vi "BELKIN EAGLE RT Main V2.vi"() -> ()   [LabVIEW 2015]
uses:
  <vilib>/vision/Image Controls.llb/IMAQ Image.ctl
  <vilib>/userdefined/High Color/IMAQdx.ctl
  Controls/BELKIN RT State.ctl
  IP results.ctl
  Controls/Command Typedef.ctl
  Stream/Controls/RT Streamer Queue element.ctl
  Stream/Controls/RT Streamer State.ctl
  Stream/LP Globals.vi
  <vilib>/FPGAPlugInAG/cRIO-9030/niLvFpga_Open_cRIO-9030.vi
  <vilib>/rvi/interface/common/dynamic/niFpgaDynamicAddResources.vi
  <vilib>/FPGAPlugInAG/Dynamic/niLvFpga_Abort_Dynamic.vi
  <vilib>/FPGAPlugInAG/Dynamic/niLvFpga_Reset_Dynamic.vi
  <vilib>/FPGAPlugInAG/Dynamic/niLvFpga_Run_Dynamic.vi
  <vilib>/Utility/error.llb/Error Cluster From Error Code.vi
  <vilib>/rvi/interface/common/niFpgaWaitOnOcc.vi
  <vilib>/rvi/errors/niLvFpgaAdjustHostInterfaceError.vi
  <vilib>/rvi/interface/nirviOpenFPGA/nirviOpenFPGA.xnode
  FPGA Bitfiles/BELKINEAGLEGUI_FPGATarget_EagleFPGAScanner_AddXN+PC+cM.lvbitx
  RT/Eagle_FPGA Scanner Control.vi
  <vilib>/rvi/interface/nirviMethod/nirviMethod.xnode
  <vilib>/rvi/interface/nirviReadWriteControl/nirviReadWriteControl.xnode
  <vilib>/rvi/interface/Simulation/niFpgaSimulationCallBeginRW.vi
  <vilib>/vision/NI_Vision_Development_Module.lvlib
  <vilib>/rvi/errors/niLvFpgaMergeErrorWithErrorCode.vi
  <vilib>/FPGAPlugInAG/Dynamic/niLvFpga_StopFifo_Dynamic.vi
  <vilib>/FPGAPlugInAG/Dynamic/niLvFpga_ConfigureFifo_Dynamic.vi
  <vilib>/FPGAPlugInAG/Dynamic/niLvFpga_StartFifo_Dynamic.vi
  NiFpgaLv.dll
panel:
  in  "FPGA VI Reference IN":refnum<k20>
  out "RoteteImages":bool
  out "Y Points":i32[](array[numeric])
  out "X Points":i32[](array[numeric])
  in  "Threshold":u8
  out "ImageIndex":i32
  out "IP Results":T1
  out "SystemState":T2=enum."Find Limbus"
  in  "Image Dir Path":path=path "c:/Images/DariaSynthMove" caption="Image Path"
  out "Simulation":bool
  in  "CamSession":T3="cam0"
  in  "AutoBalance":bool
  in  "SetParams":bool
  in  "GuiVideoRate":u8=10
  out "FrameRate":dbl
  out "EyeImage":T4
  out "Algo Time":u32
  # "Realtime Main V2"
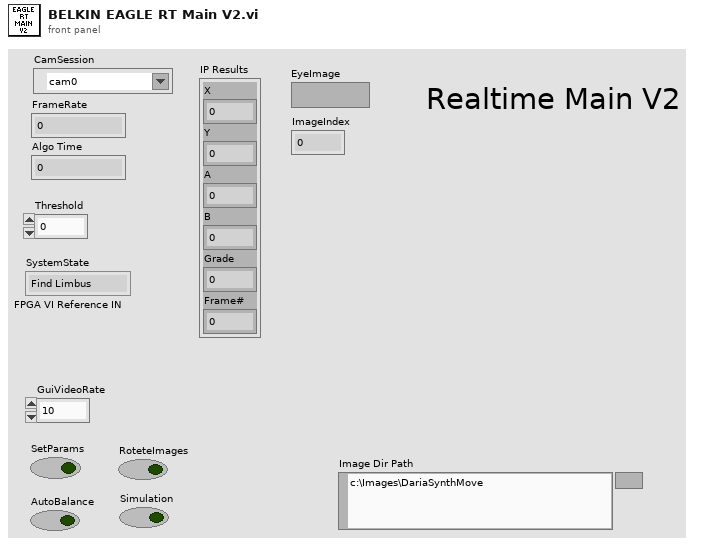
[diagram p1: front panel]
types:
  T1 = typedef "IP results.ctl" = cluster{"X":u16, "Y":u16, "A":dbl, "B":dbl, "Grade":u16, "Frame#":u16}
  T2 = typedef "BELKIN RT State.ctl" = enum16{"Initialize", "BIT", "Warm Up", "Eye Location", "Find Limbus", "Eye Track", "Fire", "Treatment Complete", "Shut Down", "Error"}
  T3 = typedef "IMAQdx.ctl" = refnum<k21>
  T4 = typedef "IMAQ Image.ctl" = refnum<image>
  T5 = typedef "Command Typedef.ctl" = cluster{"CMD":T2, "Data":variant}
  T6 = typedef "RT Streamer Queue element.ctl" = cluster{"CMD":T7, "Data":variant, "Error in":errorcluster}
  T7 = typedef "RT Streamer State.ctl" = enum16{"Init", "Idle", "Stream", "Listen", "SetRefrashRate", "SendCmdAck", "SendCmdDone", "SendSysState", "StartRecord", "Green Cordinates", "Error"}
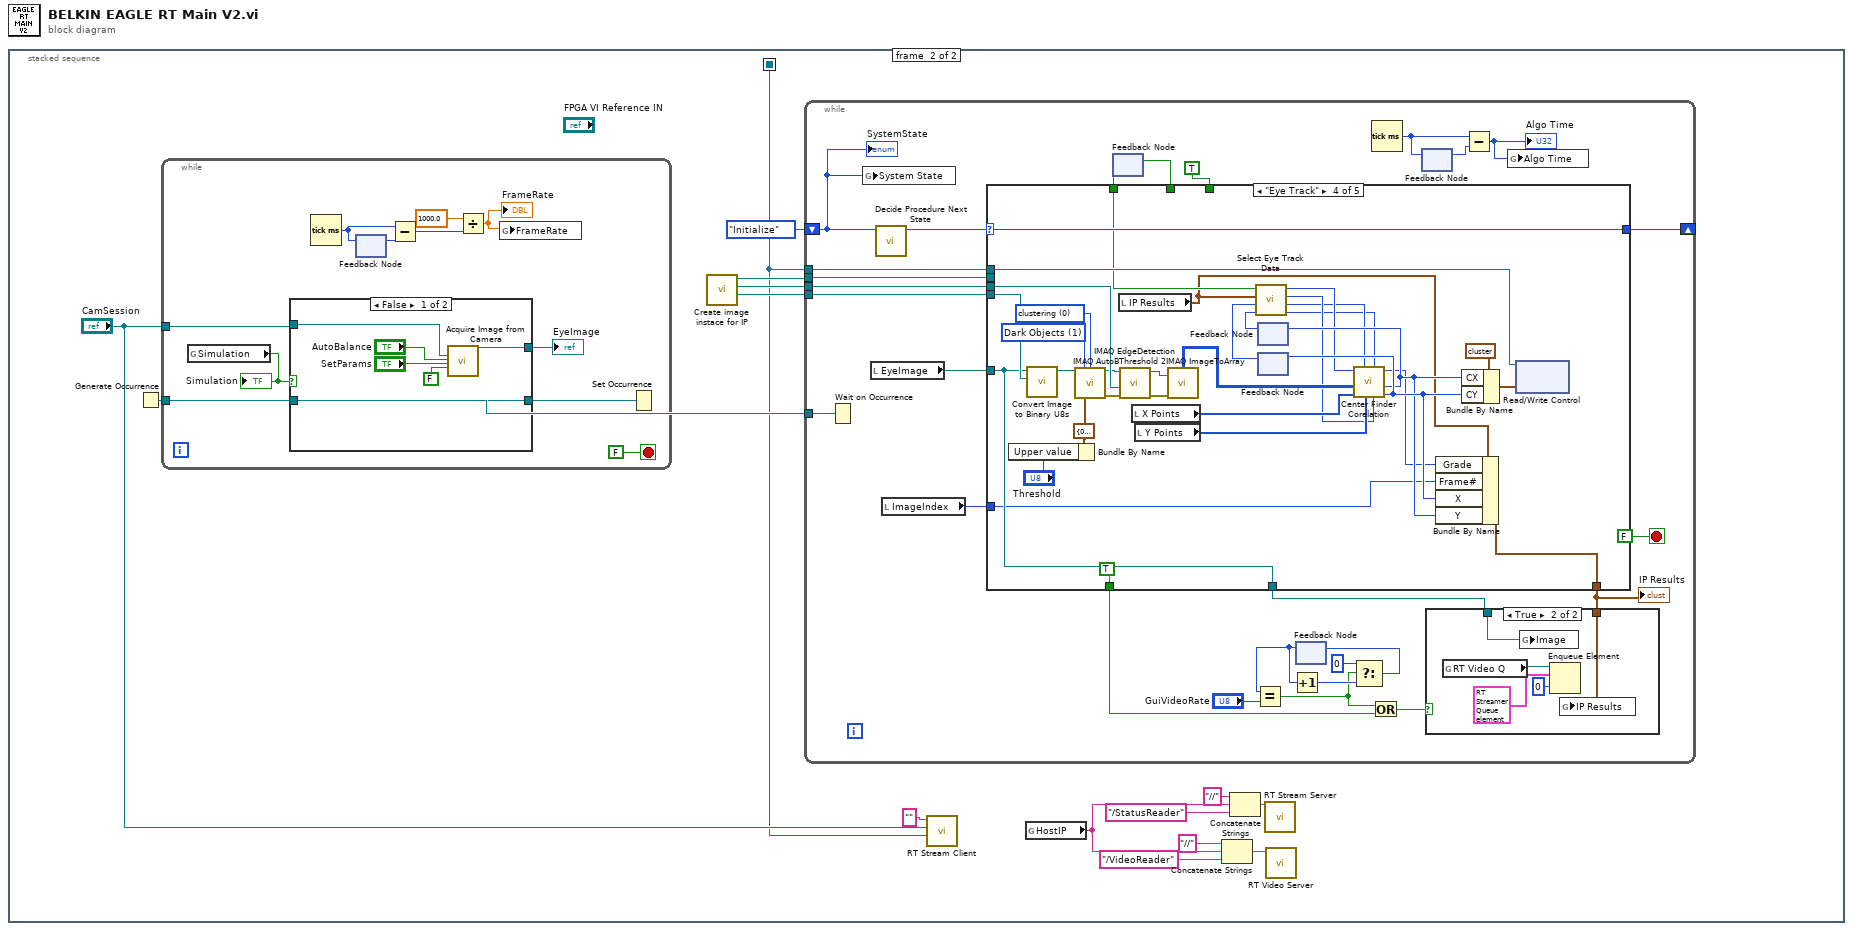
[diagram p0: block diagram]
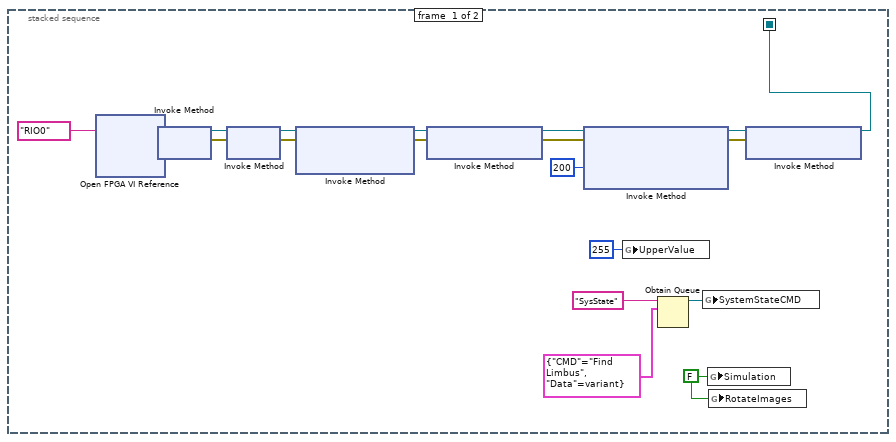
[diagram p2: hidden frame]
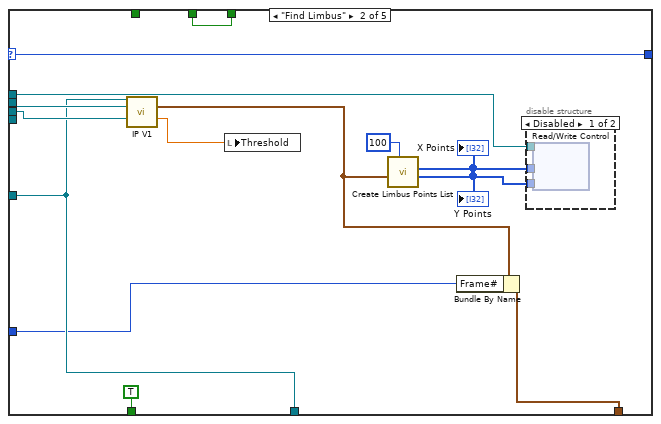
[diagram p5: hidden frame]
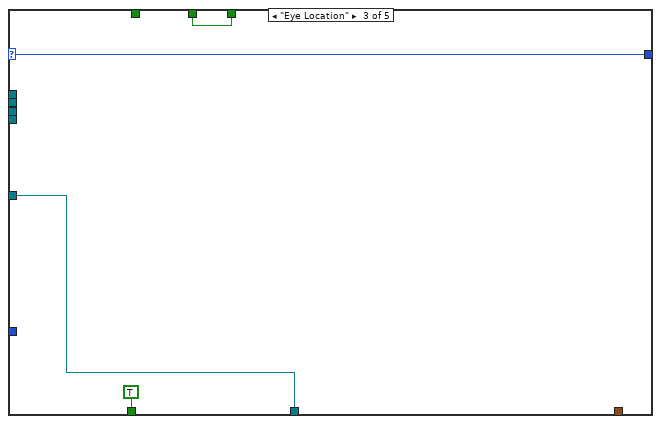
[diagram p7: hidden frame]
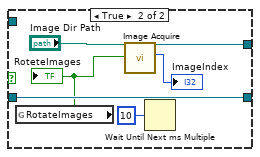
[diagram p9: hidden frame]
diagram:
  n1 = stacked-sequence {
    seq-local: [w7 _] -> [_ w21]
    frame #0 {
      w17 = FALSE ("Simulation")
      n2 = xnode "Open FPGA VI Reference"("resource name"=tag "RIO0") -> ("FPGA VI Reference Out"=w6:refnum<k20>, "error out"=w5:errorcluster)  [unwired: 1 in]
      n3 = xnode "Invoke Method"("FPGA VI Reference In"=w6, "error in"=w5) -> ("FPGA VI Reference Out"=w4:refnum<k20>, "error out"=w3:errorcluster)
      n4 = xnode "Invoke Method"("FPGA VI Reference In"=w4, "error in"=w3) -> ("FPGA VI Reference Out"=w1:refnum<k20>, "error out"=w2:errorcluster)
      n5 = xnode "Invoke Method"("FPGA VI Reference In"=w1, "error in"=w2) -> ("FPGA VI Reference Out"=w15:refnum<k20>, "error out"=w14:errorcluster)  [unwired: 1 in]
      n6 = xnode "Invoke Method"("FPGA VI Reference In"=w15, "error in"=w14) -> ("FPGA VI Reference Out"=w9:refnum<k20>, "error out"=w8:errorcluster)
      n7 = xnode "Invoke Method"("FPGA VI Reference In"=w9, "error in"=w8, "Requested Depth"=u32 200) -> ("FPGA VI Reference Out"=w11:refnum<k20>, "error out"=w10:errorcluster)  [unwired: 1 out]
      n8 = global write "LP Globals.vi" "UpperValue"(u8 255 ("UpperValue")) -> ()
      n9 = Obtain Queue(name (unnamed)="SysState", element data type=T5 {"CMD"=enum."Find Limbus", "Data"=variant}) -> (queue out=w18:refnum<queue>)  [unwired: 3 in, 2 out]
      n10 = global write "LP Globals.vi" "SystemStateCMD"(w18) -> ()
      n11 = global write "LP Globals.vi" "Simulation"(w17) -> ()
      n12 = global write "LP Globals.vi" "RotateImages"(w17) -> ()
      n13 = xnode "Invoke Method"("FPGA VI Reference In"=w11, "error in"=w10) -> ("FPGA VI Reference Out"=w7:refnum<k20>)  [unwired: 1 out]
    }
    frame #1 {
      n14 = Generate Occurrence() -> (w26:refnum<k4>)
      n15 = while {
        tunnel: "CamSession" -> [w132]
        tunnel: w26 -> [w131]
        stop <- FALSE stop-if-true
        n16 = global read "LP Globals.vi" "Simulation"() -> (w127:bool)
        "Simulation" <- w127
        n17 = case shown="False" w127 {
          tunnel: w132 -> [w143 _]
          tunnel: [w142 w149] -> w129
          tunnel: w131 -> [w141 w147]
          tunnel: [w141 w147] -> w128
          frame False {
            n18 = call "Acquire Image from Camera.vi"("Session In"=w143, "AutoBalance"="AutoBalance", "Set"="SetParams", "Stop (F)"=FALSE) -> ("Image Out"=w142:T4)  [unwired: 20 in, 3 out]
          }
          frame True {
            n19 = global read "LP Globals.vi" "RotateImages"() -> (w144:bool)
            "RoteteImages" <- w144
            n20 = call "Image Acquire.vi"("Image Dir Path"="Image Dir Path", "Next"=w144) -> ("Image Out"=w149:T4, "ImageIndex"=→"ImageIndex":i32)  [unwired: 23 in, 1 out]
            n21 = Wait Until Next ms Multiple(millisecond multiple=u32 10 ("milliseconds to wait")) -> ()  [unwired: 1 out]
          }
        }
        "EyeImage" <- w129
        n22 = Tick Count (ms)() -> (millisecond timer value=w135:u32)
        n23 = feedback-in #1(w135) -> ()
        n24 = feedback #1() -> (w134:u32)  [unwired: 1 in]
        n25 = Subtract(x=w135, y=w134) -> (x-y=w133:u32)
        n26 = Divide(x=1000.0, y=w133) -> (x/y=w130:dbl)
        "FrameRate" <- w130
        n27 = global write "LP Globals.vi" "FrameRate"(w130) -> ()
        n28 = Set Occurrence(w128) -> ()
      }
      n29 = call "Create image instace for IP.vi"() -> ("bin"=w24:T4, "Zoom"=w25:T4, "algo2"=w23:T4)  [unwired: 9 in]
      n30 = while {
        tunnel: w23 -> [w61]
        tunnel: w24 -> [w60]
        tunnel: w25 -> [w58]
        tunnel: w26 -> [w57]
        shift-right: [w54] -> _
        shift-left: BELKIN_RT_State."Initialize" ("New State") -> [w52]
        tunnel: w21 -> [w53]
        stop <- FALSE stop-if-true
        n31 = Wait on Occurrence(2:w57) -> ()  [unwired: 2 in, 1 out]
        n32 = global write "LP Globals.vi" "System State"(w52) -> ()
        n33 = local read "EyeImage"() -> (w47:T4)
        n34 = call "Decide Procedure Next State.vi"("Prev State"=w52) -> ("New State"=w51:T2)  [unwired: 9 in, 1 out]
        n35 = local read "ImageIndex"() -> (w36:i32)
        n36 = feedback #2() -> (w48:bool)  [unwired: 1 in]
        n37 = case shown="\"Eye Track\"" w51 {
          selector: w51 -> [w69 w80 w90 w121 w125]
          tunnel: w61 -> [_ w83 _ _ _]
          tunnel: w60 -> [_ _ _ w110 _]
          tunnel: w58 -> [_ w82 _ w104 _]
          tunnel: [w69 w80 w90 w121 w125] -> w54
          tunnel: w53 -> [_ w70 _ w124 _]
          tunnel: [w68 w78 w89 _ w126] -> w50
          tunnel: TRUE -> [w68 w78 w89 _ w126]
          tunnel: w48 -> [_ _ _ w112 _]
          tunnel: w47 -> [_ w77 w88 w96 _]
          tunnel: [_ w77 w88 w96 _] -> w40
          tunnel: [_ w72 _ w95 _] -> w37
          tunnel: [_ TRUE TRUE TRUE _] -> w38
          tunnel: w36 -> [_ w71 _ w92 _]
          frame "Warm Up", Default {
          }
          frame "Find Limbus" {
            n38 = call "IP V1.vi"("Image In"=w77, "Image Dst"=w83, "Zoom Image"=w82) -> ("IP Results"=w73:T1, "ThreshOut"=w79:sgl)  [unwired: 9 in, 2 out]
            n39 = local write "Threshold"(w79) -> ()
            n40 = call "Create Limbus Points List.vi"("NoOfPoints"=u16 100, "IP Results"=w73) -> ("Y Points"=w74:i16[], "X Points"=w75:i16[])  [unwired: 8 in]
            "X Points" <- w75
            "Y Points" <- w74
            n41 = Bundle By Name(cluster=w73, "Frame#"=w71) -> (w72:T1)
            n42 = disable-structure shown="Disabled" {
              disable-tunnel: w70 -> [w86 _]
              disable-tunnel: w75 -> [w85 _]
              disable-tunnel: w74 -> [w84 _]
              frame Disabled {
                n43 = xnode "Read/Write Control"("FPGA VI Reference In"=w86, "X Array"=w85, "Y Array"=w84) -> ()  [unwired: 1 in, 2 out]
              }
              frame Enabled {
              }
            }
          }
          frame "Eye Location" {
          }
          frame "Eye Track" {
            w107 = 0 items=["clustering", "entropy", "metric", "moments", "inter-class variance"] ("Method (clustering)")
            w106 = u32 1 items=["Bright Objects", "Dark Objects"] ("Look For (Bright Objects)")
            n44 = Bundle By Name(cluster=cluster{"Lower value":sgl, "Upper value":sgl} {"Lower value"=0.0, "Upper value"=255.0} ("Threshold Limits"), "Upper value"="Threshold") -> (w91:cluster{"Lower value":sgl, "Upper value":sgl})
            n45 = call "Convert Image to Binary U8s.vi"("Image Dst"=w110, "ImageIn"=w96) -> ("Image Out"=w103:T4)  [unwired: 8 in, 1 out]
            n46 = call "IMAQ AutoBThreshold 2"("Image Src"=w103, "Look For (Bright Objects)"=w106, "Method (clustering)"=w107, "Threshold Limits"=w91) -> ("Image Dst Out"=w102:T4, "error out"=w101:errorcluster)  [unwired: 9 in, 1 out]
            n47 = local read "IP Results"() -> (w93:T1)
            n48 = call "IMAQ EdgeDetection"("error in (no error)"=w101, "Image Dst"=w104, "Image Src"=w102) -> ("error out"=w111:errorcluster, "Image Dst Out"=w120:T4)  [unwired: 7 in]
            n49 = local read "X Points"() -> (w118:i32[])
            n50 = local read "Y Points"() -> (w117:i32[])
            n51 = call "IMAQ ImageToArray"("error in (no error)"=w111, "Image"=w120) -> ("Image Pixels (U8)"=w119:u8[][])  [unwired: 2 in, 4 out]
            n52 = feedback #3() -> (w116:u32)  [unwired: 1 in]
            n53 = feedback #4() -> (w115:u32)  [unwired: 1 in]
            n54 = call "Select Eye Track Data.vi"("PrevY"=w116, "PrevX"=w115, "IP Results"=w93, "ResetEyeTrack"=w112) -> ("Xmax"=w97:u32, "Ymax"=w98:u32, "Xmin"=w100:u32, "Ymin"=w99:u32)  [unwired: 4 in]
            n55 = call "Center Finder Corelation.vi"("Xmin"=w100, "Xmax"=w97, "Y_positions"=w117, "Ymax"=w98, "X_positions"=w118, "Picture"=w119, "Ymin"=w99) -> ("X"=w114:u32, "Y"=w113:u32, "Grade"=w109:u32)  [unwired: 2 in]
            n56 = feedback-in #3(w113) -> ()
            n57 = feedback-in #4(w114) -> ()
            n58 = Bundle By Name(cluster=w93, "Grade"=w109, "Frame#"=w92, "X"=w114, "Y"=w113) -> (w95:T1)
            n59 = Bundle By Name(cluster=cluster{"CX":fxp<+,10,10>, "CY":fxp<+,10,10>} {"CX"=0.0, "CY"=0.0} ("Center"), "CX"=w113, "CY"=w114) -> (w122:cluster{"CX":fxp<+,10,10>, "CY":fxp<+,10,10>})
            n60 = xnode "Read/Write Control"("FPGA VI Reference In"=w124, "Center"=w122) -> ()  [unwired: 1 in, 2 out]
          }
          frame "Fire" {
          }
        }
        "IP Results" <- w37
        n61 = feedback-in #2(w50) -> ()
        n62 = feedback #5() -> (w46:u8)  [unwired: 1 in]
        n63 = Equal?(x=w46, y="GuiVideoRate") -> (x = y?=w41:bool)
        n64 = Increment(x=w46) -> (x+1=w45:u8)
        n65 = Select(t=u8 0, s=w41, f=w45) -> (s? t:f=w44:u8)
        n66 = feedback-in #5(w44) -> ()
        n67 = Or(x=w41, y=w38) -> (x .or. y?=w39:bool)
        n68 = Tick Count (ms)() -> (millisecond timer value=w56:u32)
        n69 = feedback-in #6(w56) -> ()
        n70 = feedback #6() -> (w55:u32)  [unwired: 1 in]
        n71 = case shown="True" w39 {
          tunnel: w40 -> [_ w66]
          tunnel: w37 -> [_ w63]
          frame False {
          }
          frame True {
            n72 = global read "LP Globals.vi" "RT Video Q"() -> (w67:refnum<queue>)
            n73 = global write "LP Globals.vi" "Image"(w66) -> ()
            n74 = Enqueue Element(queue=w67, element=T6 {"CMD"=enum."Stream", "Data"=variant, "Error in"={"status"=FALSE, "code"=0, "source"=""}}, timeout in ms (-1)=0) -> ()  [unwired: 1 in, 3 out]
            n75 = global write "LP Globals.vi" "IP Results"(w63) -> ()
          }
        }
        n76 = Subtract(x=w56, y=w55) -> (x-y=w59:u32)
        "Algo Time" <- w59
        n77 = global write "LP Globals.vi" "Algo Time"(w59) -> ()
        "SystemState" <- w52
      }
      n78 = call "RT Stream Client.vi"("FPGA Reference"=w21, "CamSession"="CamSession", "Writer url"="") -> ()  [unwired: 9 in]
      n79 = global read "LP Globals.vi" "HostIP"() -> (w28:string)
      n80 = Concatenate Strings("//" ("string"), w28, "/VideoReader" ("reader url")) -> (w33:string)
      n81 = Concatenate Strings("//" ("string"), w28, "/StatusReader" ("reader url")) -> (w30:string)
      n82 = call "RT Stream Server.vi"("reader url"=w30) -> ()  [unwired: 11 in]
      n83 = call "RT Video Server.vi"("reader url"=w33) -> ()  [unwired: 11 in]
    }
  }
